vi "Eurotherm_connect.vi"() -> (0 "error out":errorcluster, 3 "Modbus Master out":refnum<class "Modbus Master.lvclass">)   [LabVIEW 2022 SP3, in "CC_Library.lvlib"]
uses:
  CC_Library.lvlib
  <vilib>/Modbus/master/Modbus Master.lvclass
  C:/Program Files (x86)/National Instruments/LabVIEW 2022/vi.lib/Modbus/subvis/Modbus API/Modbus API.lvclass
  <vilib>/Modbus/subvis/Modbus API/Modbus API.lvclass/Modbus API.ctl
  <vilib>/Modbus/subvis/Transmission Data Unit (ADU)/Transmission Data Unit/Transmission Data Unit.lvclass/Transmission Data Unit.ctl
  <vilib>/Modbus/master/Data Access/Unit ID/Set Unit ID Property.vi
  <vilib>/Modbus/subvis/Transmission Data Unit (ADU)/Transmission Data Unit/Data Access/Unit ID/Write Unit ID.vi
  <vilib>/Modbus/subvis/Modbus API/Read Transmission Data Unit.vi
  <vilib>/Modbus/subvis/Modbus API/Write Transmission Data Unit.vi
  <vilib>/Modbus/master/Create Master Instance (TCP).vi
  <vilib>/Modbus/subvis/Transmission Data Unit (ADU)/Transmission Data Unit/Transmission Data Unit.lvclass
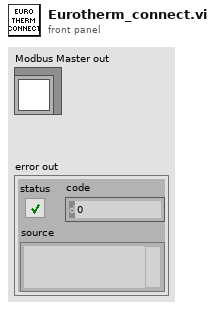
[diagram p1: front panel]
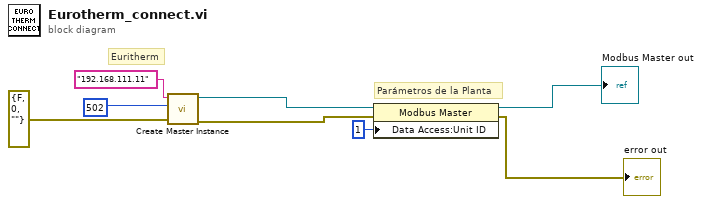
[diagram p0: block diagram]
diagram:
  # "Parámetros de la Planta"
  # "Euritherm"
  n1 = call-poly <vilib>:"Create Master Instance.vi"("error in (no error)"=errorcluster {"status"=FALSE, "code"=0, "source"=""}, "port (502)"=u16 502, "address"="192.168.111.11") -> ("error out"=w3:errorcluster, "TCP master instance"=w4:refnum<class "Modbus Master.lvclass">)  [unwired: 7 in]
  n2 = property class="Modbus Master"(reference=w4, error in=w3, "Data Access:Unit ID"=u8 1 ("Unit ID")) -> (reference out=→"Modbus Master out":refnum<class "Modbus Master.lvclass">, error out=→"error out":errorcluster)
